vi "Draw Image from File.vi"(8 "error in (no error)":errorcluster, 9 "top left (0,0)":cluster{"x":i16, "y":i16}, 10 "picture":picture, 11 "path to BMP file":path) -> (0 "error out":errorcluster, 1 "image size (pixels)":cluster{"x":i16, "y":i16}, 2 "new picture":picture, 3 "dup path":path)   [LabVIEW 2009]
doc: "Reads a BMP, JPG or PNG file and draws it into a picture control."
uses:
  <userlib>/_OpenG.lib/file/file.llb/Strip Path Extension - Path__ogtk.vi
panel:
  # "[OpenG VI Tags] ***Do Not Remove***"
  # "Draw Image From File.vi\n\nReads a BMP, JPG or PNG file and draws it into a picture control.\n\nPlease visit http://www.OpenG.org to learn about the\nOpen Source LabVIEW software movement.\n\nNOTICE -- YOU MUST LEAVE THIS NOTICE IN PLACE.  PER THE TERMS OF THE LICENSE BELOW, YOU MAY SUBLICENSE THIS SOFTWARE \nIN ANY WAY THAT DOES NOT CONFLICT WITH THIS LICENSE.\n\n### BSD License (http://www.opensource.org/licenses/bsd-license.php) Begin ###\n\nCopyright (c) 2006, JKI <info@jameskring.com>; Authors:  Jim Kring <jim@jimkring.com>, Philippe Guerit <pjm_labview@yahoo.com>\nCopyright (c) 2002, Jim Kring <jim@jimkring.com>\nCopyright (c) 2002, Rolf Kalbermatter <rolf.kalbermatter@citeng.com>\nCopyright (c) 2007, Bill Clench <bclench@yahoo.com>\n\nAll rights reserved.\n\nRedistribution and use in source and binary forms, with or without modification, are permitted provided that the following conditions are met:\n\n    * Redistributions of source code must retain the above copyright notice, this list of conditions and the following disclaimer.\n    * Redistributions in binary form must reproduce the above copyright notice, this list of conditions and the following disclaimer in the \n       documentation and/or other materials provided with the distribution.\n    * Neither the name of SciWare, James Kring, Inc., nor the names of its contributors may be used to endorse or promote products derived \n       from this software without specific prior written permission.\n\nTHIS SOFTWARE IS PROVIDED BY THE COPYRIGHT HOLDERS AND CONTRIBUTORS \"AS IS\" AND ANY EXPRESS OR IMPLIED WARRANTIES, \nINCLUDING, BUT NOT LIMITED TO, THE IMPLIED WARRANTIES OF MERCHANTABILITY AND FITNESS FOR A PARTICULAR PURPOSE ARE \nDISCLAIMED. IN NO EVENT SHALL THE COPYRIGHT OWNER OR CONTRIBUTORS BE LIABLE FOR ANY DIRECT, INDIRECT, INCIDENTAL,\n SPECIAL, EXEMPLARY, OR CONSEQUENTIAL DAMAGES (INCLUDING, BUT NOT LIMITED TO, PROCUREMENT OF SUBSTITUTE GOODS OR \nSERVICES; LOSS OF USE, DATA, OR PROFITS; OR BUSINESS INTERRUPTION) HOWEVER CAUSED AND ON ANY THEORY OF LIABILITY, \nWHETHER IN CONTRACT, STRICT LIABILITY, OR TORT (INCLUDING NEGLIGENCE OR OTHERWISE) ARISING IN ANY WAY OUT OF THE USE \nOF THIS SOFTWARE, EVEN IF ADVISED OF THE POSSIBILITY OF SUCH DAMAGE.\n\n### BSD License End ###"
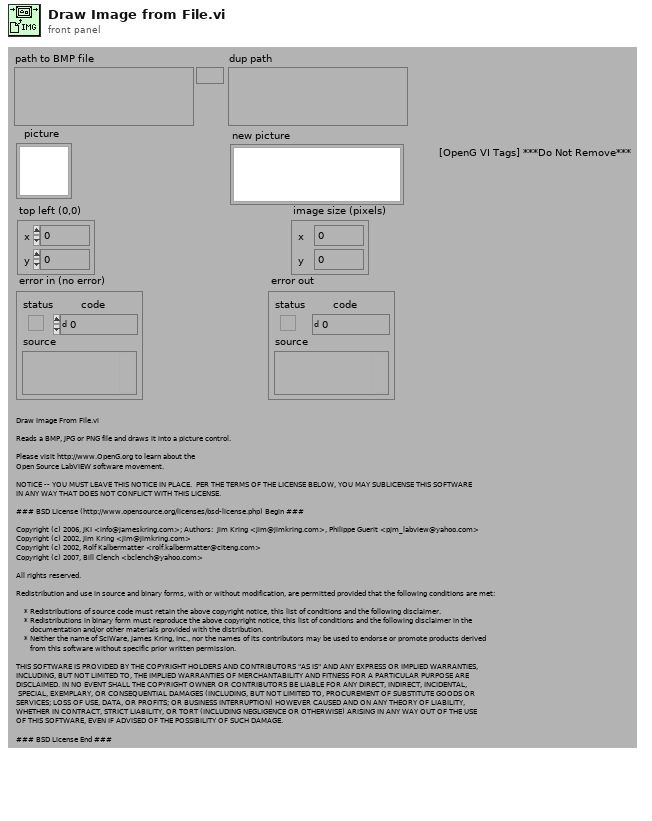
[diagram p1: front panel]
types:
  T1 = cluster{"left":i16, "top":i16, "right":i16, "bottom":i16}
  T2 = typedef "imagedata.ctl" = cluster{"image type":i32, "image depth":i32, "image":u8[], "mask":u8[], "colors":u32[], "Rectangle":cluster{"left":i16, "top":i16, "right":i16, "bottom":i16}}
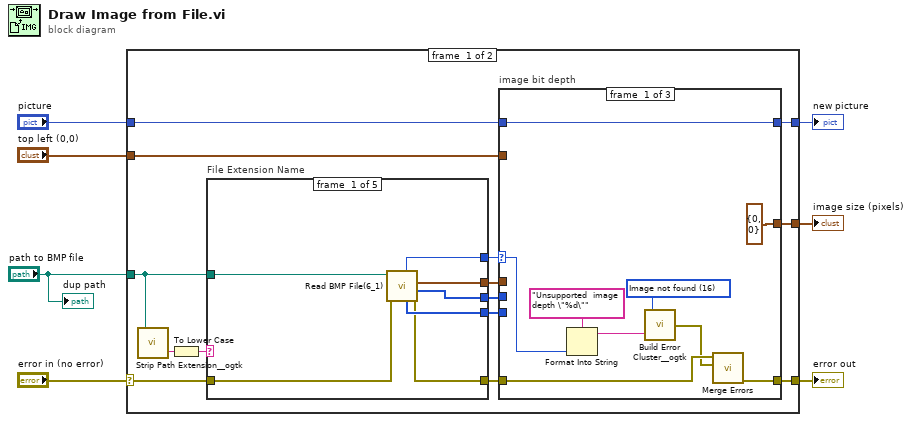
[diagram p0: block diagram]
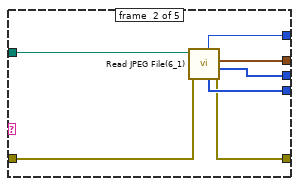
[diagram p2: hidden frame]
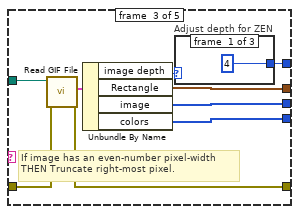
[diagram p3: hidden frame]
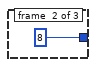
[diagram p4: hidden frame]
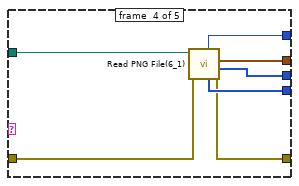
[diagram p6: hidden frame]
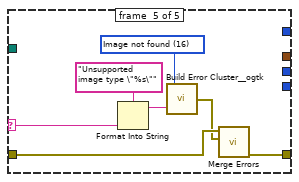
[diagram p7: hidden frame]
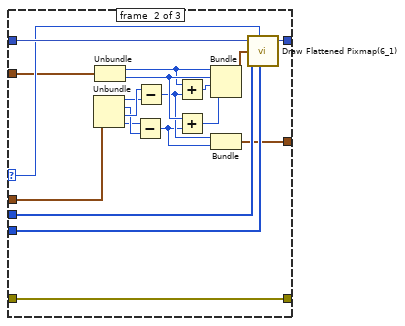
[diagram p8: hidden frame]
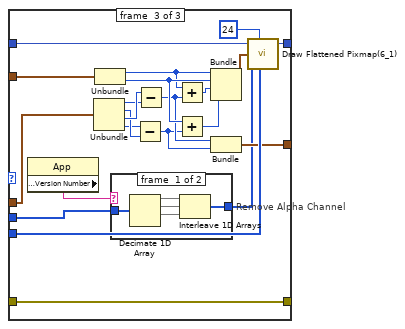
[diagram p9: hidden frame]
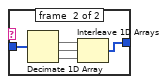
[diagram p10: hidden frame]
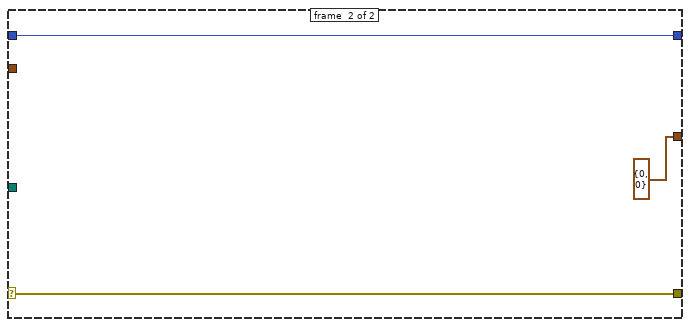
[diagram p11: hidden frame]
diagram:
  n1 = case shown="No Error" "error in (no error)" {
    selector: "error in (no error)" -> [w16 w125]
    tunnel: "path to BMP file" -> [w10 _]
    tunnel: "picture" -> [w21 w124]
    tunnel: [w20 w124] -> w6
    tunnel: [w17 cluster{i16, i16} {0, 0}] -> w5
    tunnel: [w14 w125] -> w3
    tunnel: "top left (0,0)" -> [w13 _]
    frame #0 {
      n2 = call-poly <userlib>:"Strip Path Extension__ogtk.vi"("path"=w10) -> ("extension"=w9:string)  [unwired: 1 out]
      n3 = To Lower Case(string=w9) -> (all lower case string=w8:string)
      n4 = case "File Extension Name" shown="\"gif\"" w8 {
        selector: w8 -> [_ _ _ _ w60]
        tunnel: [w28 w35 w40 w54 _] -> w19
        tunnel: [w27 w34 w42 w53 _] -> w18
        tunnel: w16 -> [w26 w33 w39 w52 w57]
        tunnel: [w25 w32 w38 w51 w55] -> w15
        tunnel: [w24 w31 w44 w50 _] -> w12
        tunnel: [w23 w30 w43 w49 _] -> w11
        tunnel: w10 -> [w22 w29 w37 w48 _]
        frame #0 {
          n5 = call <vilib>:"Read BMP File(6_1).vi"("error in (no error)"=w26, "path to BMP file"=w22) -> ("error out"=w25:errorcluster, "flattened image data"=w23:u8[], "rect"=w24:T1, "color table"=w27:u32[], "depth"=w28:u8)  [unwired: 4 in, 1 out]
        }
        frame #1 {
          n6 = call <vilib>:"Read JPEG File(6_1).vi"("error in (no error)"=w33, "path to JPEG file"=w29) -> ("error out"=w32:errorcluster, "flattened image data"=w30:u8[], "rect"=w31:T1, "colorTable"=w34:u32[], "depth"=w35:u8)  [unwired: 4 in, 1 out]
        }
        frame #2 {
          # "If image has an even-number pixel-width\nTHEN Truncate right-most pixel."
          n7 = call "Read GIF File.vi"("error in (no error)"=w39, "path to GIF file"=w37) -> ("error out"=w38:errorcluster, "image data"=w36:T2)  [unwired: 7 in, 1 out]
          n8 = Unbundle By Name(w36) -> ("image depth"=w41:i32, "Rectangle"=w44:T1, "image"=w43:u8[], "colors"=w42:u32[])
          n9 = case "Adjust depth for ZEN" shown="Default" w41 {
            selector: w41 -> [_ _ w47]
            tunnel: [4 8 w47] -> w40
            frame #0 {
            }
            frame #1 {
            }
            frame #2 {
            }
          }
        }
        frame #3 {
          n10 = call <vilib>:"Read PNG File(6_1).vi"("error in (no error)"=w52, "path to PNG file"=w48) -> ("error out"=w51:errorcluster, "flattened image data"=w49:u8[], "rect"=w50:T1, "colorTable"=w53:u32[], "depth"=w54:u8)  [unwired: 4 in, 1 out]
        }
        frame #4 {
          w61 = 16 items=["No error", "Argument error", "Memory is full", "Out of zone", "End of file", "File already open", "Generic file I/O error", "File not found", "File permission error", "Disk is full", "Duplicate path", "Too many files open", "System feature not enabled", "Resource file not found", "Cannot add resource", "Resource not found", "Image not found", "Image memory error", "Pen does not exist", "Config type invalid", "Config token not found", "Config parse error", "Config memory error", "Bad external code format", "Bad external code offset", "External code not present", "Null window", "Destroy window error", "Null menu", "Print aborted", "Bad print record", "Print driver error", "Windows error during printing", "Memory error during printing", "Print dialog error", "Generic print error", "Invalid device refnum", "Device not found", "Device parameter error", "Device unit error", "Cannot open device", "Device call aborted", "Generic error", "Cancelled by user", "Object ID too low", "Object ID too high", "Object not in heap", "Unknown heap", "Unknown object (invalid DefProc)", "Unknown object (DefProc not in table)", "Message out of range", "Invalid (null) method", "Unknown message", "Manager call not supported", "Bad address", "Network operation in progress", "Network operation timed out", "Connection is busy", "Network attribute not supported", "Network error", "Address in use", "System out of memory", "Connection aborted", "Connection refused", "Not connected", "Already connected", "Connection closed", "Initialization error (interapplication manager)", "Bad occurrence", "Wait on unbound occurrence handler", "Occurrence queue overflow", "Datalog type conflict", "Unused", "Unrecognized type (interapplication manager)", "Memory corrupt", "Failed to make temporary DLL", "Old CIN version", "Drag socket not found", "Failed to load drop-object", "Failed to register OLE object", "Failed to release OLE object", "Format specifier type mismatch", "Unknown format specifier", "Too few format specifiers", "Too many format specifiers", "Scan failed", "Newer CIN version", "Error converting to variant", "Runtime menu error", "Password tampered", "Variant attribute not found", "Incompatible variant data type", "Event data is not available", "Event Store is not present", "Occurrence is not found", "Event Queue is not created", "Event info is not available", "Refnum passed is NULL", "Error retrieving Class GUID", "Error retrieving CoClass GUID", "Error retrieving TypeLib GUID.", "Bad built application magic bytes.", "Specific driver is different from the specific driver associated with the Logical Name.", "There is no session opened to the class driver.", "Max Error", "MAX - Error with config objects", "MAX - Error loading configuration", "MAX - Group not supported"]
          n11 = Format Into String(format string="Unsupported image type \"%s\"" ("String to Prepend to source (\"\")"), w60) -> (resulting string=w58:string)  [unwired: 2 in, 1 out]
          n12 = call <userlib>:"Build Error Cluster__ogtk.vi"("String to Prepend to source (\"\")"=w58, "code"=w61) -> ("error out"=w56:errorcluster)
          n13 = call <vilib>:"Merge Errors.vi"("error in 2 (no error)"=w56, "error in 1 (no error)"=w57) -> ("error out"=w55:errorcluster)  [unwired: 5 in]
        }
      }
      n14 = case "image bit depth" shown="1, 4, 8, 24" w19 {
        selector: w19 -> [w63 w85 _]
        tunnel: w21 -> [w70 w90 w112]
        tunnel: [w70 w89 w111] -> w20
        tunnel: [cluster{i16, i16} {0, 0} w80 w104] -> w17
        tunnel: w18 -> [_ w86 w109]
        tunnel: w15 -> [w67 w88 w110]
        tunnel: [w65 w88 w110] -> w14
        tunnel: w13 -> [_ w72 w96]
        tunnel: w12 -> [_ w79 w103]
        tunnel: w11 -> [_ w87 w93]
        frame #0 {
          w68 = 16 items=["No error", "Argument error", "Memory is full", "Out of zone", "End of file", "File already open", "Generic file I/O error", "File not found", "File permission error", "Disk is full", "Duplicate path", "Too many files open", "System feature not enabled", "Resource file not found", "Cannot add resource", "Resource not found", "Image not found", "Image memory error", "Pen does not exist", "Config type invalid", "Config token not found", "Config parse error", "Config memory error", "Bad external code format", "Bad external code offset", "External code not present", "Null window", "Destroy window error", "Null menu", "Print aborted", "Bad print record", "Print driver error", "Windows error during printing", "Memory error during printing", "Print dialog error", "Generic print error", "Invalid device refnum", "Device not found", "Device parameter error", "Device unit error", "Cannot open device", "Device call aborted", "Generic error", "Cancelled by user", "Object ID too low", "Object ID too high", "Object not in heap", "Unknown heap", "Unknown object (invalid DefProc)", "Unknown object (DefProc not in table)", "Message out of range", "Invalid (null) method", "Unknown message", "Manager call not supported", "Bad address", "Network operation in progress", "Network operation timed out", "Connection is busy", "Network attribute not supported", "Network error", "Address in use", "System out of memory", "Connection aborted", "Connection refused", "Not connected", "Already connected", "Connection closed", "Initialization error (interapplication manager)", "Bad occurrence", "Wait on unbound occurrence handler", "Occurrence queue overflow", "Datalog type conflict", "Unused", "Unrecognized type (interapplication manager)", "Memory corrupt", "Failed to make temporary DLL", "Old CIN version", "Drag socket not found", "Failed to load drop-object", "Failed to register OLE object", "Failed to release OLE object", "Format specifier type mismatch", "Unknown format specifier", "Too few format specifiers", "Too many format specifiers", "Scan failed", "Newer CIN version", "Error converting to variant", "Runtime menu error", "Password tampered", "Variant attribute not found", "Incompatible variant data type", "Event data is not available", "Event Store is not present", "Occurrence is not found", "Event Queue is not created", "Event info is not available", "Refnum passed is NULL", "Error retrieving Class GUID", "Error retrieving CoClass GUID", "Error retrieving TypeLib GUID.", "Bad built application magic bytes.", "Specific driver is different from the specific driver associated with the Logical Name.", "There is no session opened to the class driver.", "Max Error", "MAX - Error with config objects", "MAX - Error loading configuration", "MAX - Group not supported"]
          n15 = Format Into String(format string="Unsupported  image depth \"%d\"" ("String to Prepend to source (\"\")"), w63) -> (resulting string=w62:string)  [unwired: 2 in, 1 out]
          n16 = call <userlib>:"Build Error Cluster__ogtk.vi"("String to Prepend to source (\"\")"=w62, "code"=w68) -> ("error out"=w66:errorcluster)
          n17 = call <vilib>:"Merge Errors.vi"("error in 2 (no error)"=w66, "error in 1 (no error)"=w67) -> ("error out"=w65:errorcluster)  [unwired: 5 in]
        }
        frame #1 {
          n18 = Unbundle(w79) -> ("left"=w83:i16, "top"=w82:i16, "right"=w84:i16, "bottom"=w81:i16)
          n19 = Unbundle(w72) -> ("x"=w74:i16, "y"=w76:i16)
          n20 = Subtract(x=w81, y=w82) -> (x-y=w73:i16)
          n21 = Subtract(x=w84, y=w83) -> (x-y=w75:i16)
          n22 = Add(x=w74, y=w75) -> (x+y=w78:i16)
          n23 = Add(x=w76, y=w73) -> (x+y=w77:i16)
          n24 = Bundle("x"=w74, "y"=w76, w78, w77) -> (w71:cluster{"x":i16, "y":i16, i16, i16})  [unwired: 1 in]
          n25 = Bundle(w75, w73) -> (w80:cluster{i16, i16})  [unwired: 1 in]
          n26 = call <vilib>:"Draw Flattened Pixmap(6_1).vi"("picture"=w90, "bit depth(8)"=w85, "rect"=w71, "flattened pixmap data"=w87, "color table"=w86) -> ("new picture"=w89:picture)  [unwired: 4 in]
        }
        frame #2 {
          n27 = property class="App"() -> ("Application:Version Number"=w91:string)  [unwired: 2 in, 2 out]
          n28 = Unbundle(w103) -> ("left"=w107:i16, "top"=w106:i16, "right"=w108:i16, "bottom"=w105:i16)
          n29 = Unbundle(w96) -> ("x"=w98:i16, "y"=w100:i16)
          n30 = case "Remove Alpha Channel" shown="Default" w91 {
            tunnel: w93 -> [w117 w122]
            tunnel: [w114 w119] -> w92
            frame #0 {
              n31 = Decimate 1D Array(w117) -> (w113:u8[], w115:u8[], w116:u8[])  [unwired: 1 out]
              n32 = Interleave 1D Arrays(w113, w115, w116) -> (w114:u8[])
            }
            frame #1 {
              n33 = Decimate 1D Array(w122) -> (w120:u8[], w121:u8[], w118:u8[])  [unwired: 1 out]
              n34 = Interleave 1D Arrays(w120, w121, w118) -> (w119:u8[])
            }
          }
          n35 = Subtract(x=w105, y=w106) -> (x-y=w97:i16)
          n36 = Subtract(x=w108, y=w107) -> (x-y=w99:i16)
          n37 = Add(x=w98, y=w99) -> (x+y=w102:i16)
          n38 = Add(x=w100, y=w97) -> (x+y=w101:i16)
          n39 = Bundle("x"=w98, "y"=w100, w102, w101) -> (w95:cluster{"x":i16, "y":i16, i16, i16})  [unwired: 1 in]
          n40 = Bundle(w99, w97) -> (w104:cluster{i16, i16})  [unwired: 1 in]
          n41 = call <vilib>:"Draw Flattened Pixmap(6_1).vi"("picture"=w112, "bit depth(8)"=u8 24, "rect"=w95, "flattened pixmap data"=w92, "color table"=w109) -> ("new picture"=w111:picture)  [unwired: 4 in]
        }
      }
    }
    frame #1 {
    }
  }
  "new picture" <- w6
  "image size (pixels)" <- w5
  "error out" <- w3
  "dup path" <- "path to BMP file"
